vi "2D Cross Correlation (DBL).vi"(8 "algorithm":enum32{"direct", "frequency domain"}(ring)=enum."frequency domain", 10 "Y":dbl[][](array[numeric]), 11 "X":dbl[][](array[numeric])) -> (0 "error":i32, 3 "Rxy":dbl[][](array[numeric]))   [LabVIEW 2020, in "NI_AALPro.lvlib"]
doc: "Computes the cross correlation of the input sequences <B>X</B> and <B>Y</B>. Wire data to the <B>X</B> and <B>Y</B> inputs to determine the polymorphic instance to use or manually select the instance."
uses:
  NI_AALPro.lvlib
  <resource>/lvanlys.dll
panel:
  # "2D CrossCorrelation (DBL)"
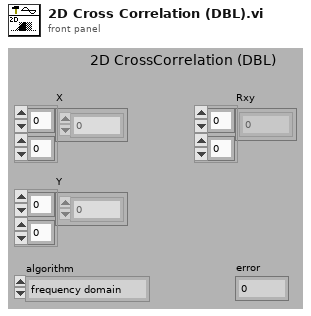
[diagram p1: front panel]
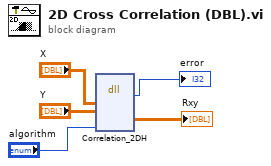
[diagram p0: block diagram]
diagram:
  n1 = dll-call lib="C:/Program Files (x86)/National Instruments/LabVIEW 2020/resource/lvanlys.*" fn="Correlation_2DH"("xH"="X", "yH"="Y", "domain"="algorithm") -> (→"error":i32, "rxyH"=→"Rxy":dbl[][])  [unwired: 7 in, 2 out]
